vi "ScopeCheck.vi"() -> ()   [LabVIEW 2011]
uses:
  <vilib>/measure/matone.llb/Extract Single Tone Information N Chan.vi
  <vilib>/measure/NI_MAPro.lvlib
panel:
  out "STFT Spectrogram 3":dbl[][](graph)
  out "STFT Spectrogram 2":dbl[][](graph)
  out "STFT Spectrogram":dbl[][](graph)
  in  "stop":bool
  out "Waveform Chart":dbl[][](graph)
  out "signal":dynamicdata(graph)
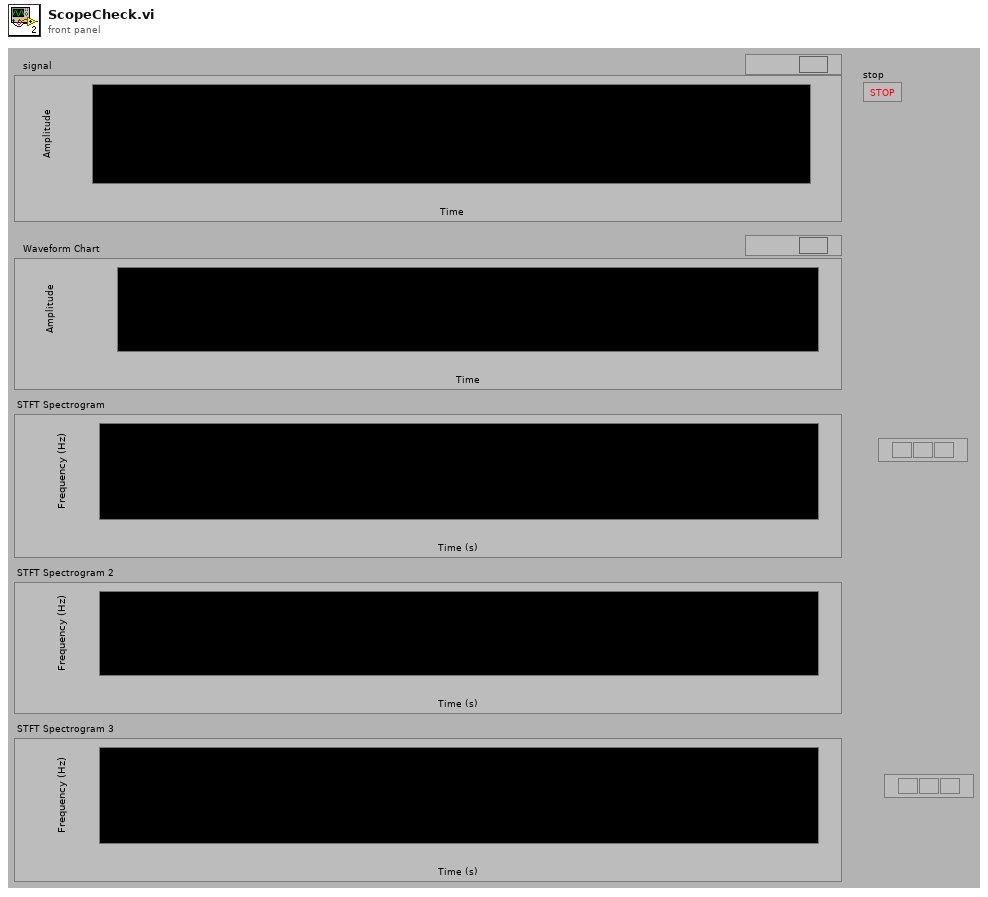
[diagram p1: front panel]
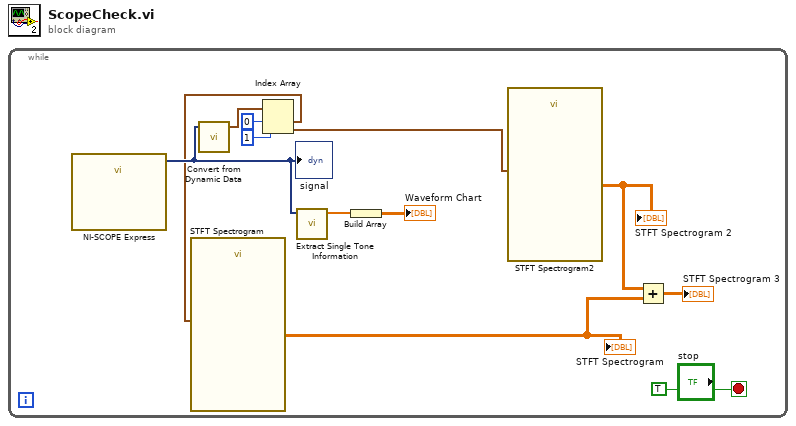
[diagram p0: block diagram]
diagram:
  n1 = while {
    stop <- TRUE stop-if-true
    n2 = call "NI-SCOPE Express"() -> ("signal"=w10:dynamicdata)  [unwired: 3 in, 12 out]
    "signal" <- w10
    n3 = call "Convert from Dynamic Data"("Dynamic Data Type"=w10) -> ("Array of Waveform"=w9:waveform(dbl)[])  [unwired: 3 out]
    n4 = Index Array(array=w9, index #1=0 ("index"), index #2=1 ("index")) -> (element #1=w5:waveform(dbl), element #2=w6:waveform(dbl))
    n5 = call "STFT Spectrogram"("Signal"=w5) -> ("Spectrogram"=w3:dbl[][])  [unwired: 2 in, 8 out]
    "STFT Spectrogram" <- w3
    n6 = call-poly <vilib>:"Extract Single Tone Information.vi"("time signals in"=w10) -> ("detected frequencies"=w12:dbl[])  [unwired: 3 in, 7 out]
    n7 = Build Array(w12) -> (→"Waveform Chart":dbl[][])
    n8 = call "STFT Spectrogram2"("Signal"=w6) -> ("Spectrogram"=w4:dbl[][])  [unwired: 2 in, 8 out]
    "STFT Spectrogram 2" <- w4
    n9 = Add(x=w4, y=w3) -> (x+y=→"STFT Spectrogram 3":dbl[][])
  }
